vi "Write ActiveFlag.vi"(8 "error in (no error)":errorcluster, 10 "ActiveFlag":cluster{"Axis 1":T1, "Axis 2":T1, "Axis 3":T1}, 11 "ESP301 in":refnum<class "ESP301.lvclass">) -> (0 "error out":errorcluster, 3 "ESP301 out":refnum<class "ESP301.lvclass">)   [LabVIEW 2020, in "ESP301.lvclass"]
uses:
  ESP301.lvclass
  activeflag.ctl
  ESP301.lvclass/ESP301.ctl
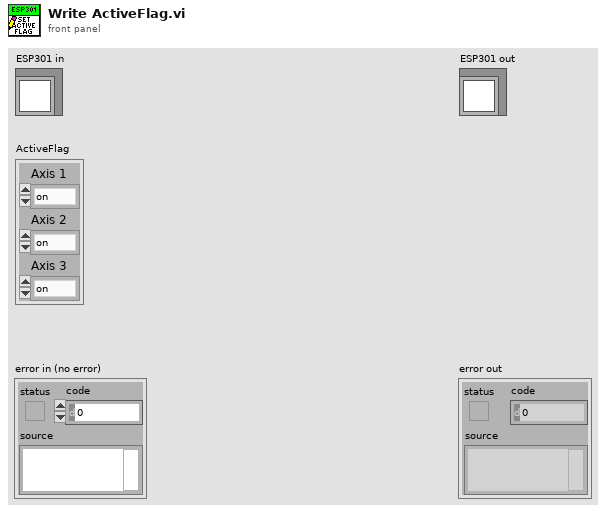
[diagram p1: front panel]
types:
  T1 = typedef "activeflag.ctl" = enum16{"on", "off", "n/a"}
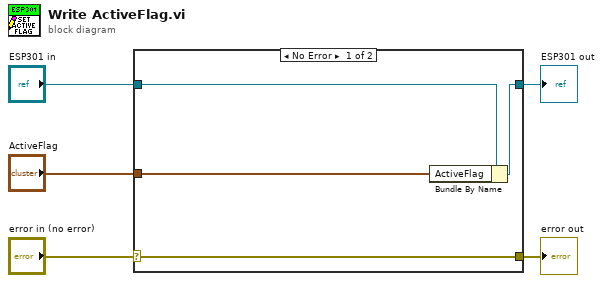
[diagram p0: block diagram]
diagram:
  n1 = case shown="No Error" "error in (no error)" {
    selector: "error in (no error)" -> [w9 w10]
    tunnel: [w9 w10] -> w4
    tunnel: [w7 w11] -> w2
    tunnel: "ESP301 in" -> [w8 w11]
    tunnel: "ActiveFlag" -> [w6 _]
    frame No Error {
      n2 = Bundle By Name(cluster=w8, "ActiveFlag"=w6) -> (w7:refnum<class "ESP301.lvclass">)
    }
    frame Error {
    }
  }
  "error out" <- w4
  "ESP301 out" <- w2
